vi "GetDescription.vi"(8 "Error In":errorcluster, 11 "reference in":refnum<class "UnderlineDecorator.lvclass">) -> (0 "Error Out":errorcluster, 2 "Description":string, 3 "reference out":refnum<class "UnderlineDecorator.lvclass">)   [LabVIEW 2024, in "UnderlineDecorator.lvclass"]
uses:
  UnderlineDecorator.lvclass
  IText/IText.lvclass
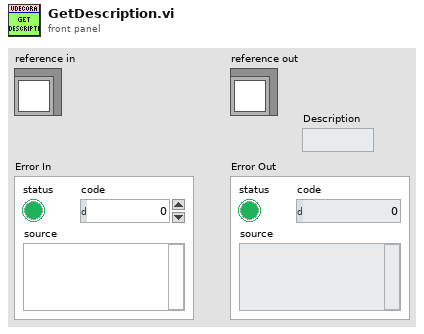
[diagram p1: front panel]
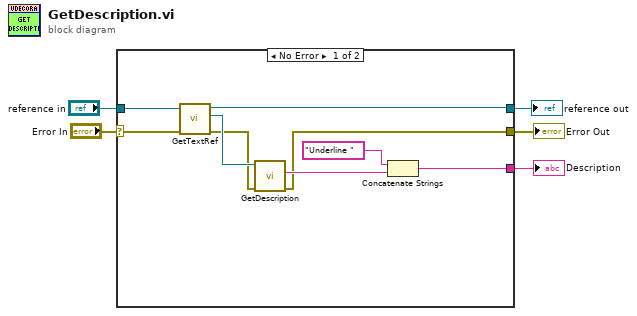
[diagram p0: block diagram]
diagram:
  n1 = case shown="No Error" "Error In" {
    selector: "Error In" -> [w14 w16]
    tunnel: [w6 w16] -> w4
    tunnel: [w12 w15] -> w2
    tunnel: "reference in" -> [w13 w15]
    tunnel: [w8 _] -> w1
    frame No Error {
      n2 = call-dynamic "GetTextRef.vi"("Error In"=w14, "reference in"=w13) -> ("Error Out"=w7:errorcluster, "TextRef"=w11:refnum<class "IText.lvclass">, "reference out"=w12:refnum<class "UnderlineDecorator.lvclass">)  [unwired: 7 in]
      n3 = call-dynamic "GetDescription.vi"("Error In"=w7, "object in"=w11) -> ("Error Out"=w6:errorcluster, "Description"=w10:string)  [unwired: 7 in, 1 out]
      n4 = Concatenate Strings("Underline " ("string"), w10) -> (w8:string)
    }
    frame Error {
    }
  }
  "Error Out" <- w4
  "reference out" <- w2
  "Description" <- w1
